vi "LeftClick.vi"(8 "Error in (no error)":errorcluster, 11 "Click?":bool=TRUE) -> (0 "Error out":errorcluster)   [LabVIEW 2013]
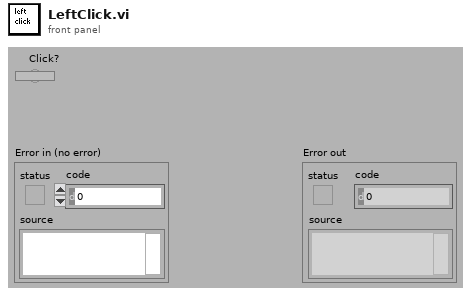
[diagram p1: front panel]
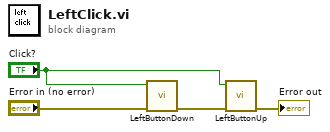
[diagram p0: block diagram]
diagram:
  n1 = call "LeftButtonDown.vi"("Error in (no error)"="Error in (no error)", "Click?"="Click?") -> ("Error out"=w4:errorcluster)  [unwired: 9 in]
  n2 = call "LeftButtonUp.vi"("Error in (no error)"=w4, "Click?"="Click?") -> ("Error out"=→"Error out":errorcluster)  [unwired: 9 in]
